vi "AFT Create FIR QR-RLS.vi"   [LabVIEW 2017, in "NI_AdaptiveFilter.lvlib"]
doc: "Creates a finite impulse response (FIR) adaptive filter with the QR decomposition-based recursive least squares (QR-RLS) algorithm. You must manually select the polymorphic instance you want to use."
uses:
  <vilib>/addons/Adaptive Filters/NI_AdaptiveFilter.lvlib
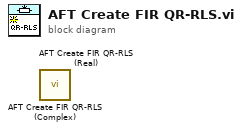
[diagram p0: block diagram]
diagram:
  n1 = call <vilib>:"AFT Create FIR QR-RLS (Complex).vi"() -> ()  [unwired: 10 in, 2 out]
  n2 = call <vilib>:"AFT Create FIR QR-RLS (Real).vi"() -> ()  [unwired: 10 in, 2 out]
